vi "G2CPU Not Complex Process.vi"(10 "Backend":T1 items=["Default Backend"=0, "CPU Backend"=1, "CUDA Backend"=2, "OPENCL Backend"=4, "Intel OneAPI"=8], 11 "X size":i32=16384) -> (3 "G2CPU Time":dbl)   [LabVIEW 2020]
uses:
  <vilib>/Natan Biesmans/G2CPU GPU and CPU HPC Toolkit/ArrayFire Driver/TypeDefs/backend.ctl
  fbbaf97c-3b5e-4b4c-bc14-40c3526c788b.vi
  c2200195-6f6b-46fb-afe8-d4cd0bcb91cf.vi
  fbbaf97c-3b5e-4b4c-bc14-40c3526c788b.vi/caaf1833-0905-411b-a9ed-2cc30d41907c.vi
  <vilib>/Natan Biesmans/G2CPU GPU and CPU HPC Toolkit/G2CPU Libraries/Arrays/SubVI/Array Sizes to Dim Cluster.vi
  c2200195-6f6b-46fb-afe8-d4cd0bcb91cf.vi/caaf1833-0905-411b-a9ed-2cc30d41907c.vi
  fbbaf97c-3b5e-4b4c-bc14-40c3526c788b.vi/caaf1833-0905-411b-a9ed-2cc30d41907c.vi/1a23f98f-393f-4176-8983-7f1ab824c539.vi
  c2200195-6f6b-46fb-afe8-d4cd0bcb91cf.vi/caaf1833-0905-411b-a9ed-2cc30d41907c.vi/1a23f98f-393f-4176-8983-7f1ab824c539.vi
  <vilib>/Natan Biesmans/G2CPU GPU and CPU HPC Toolkit/G2CPU Libraries/Arrays/1DArray/f32/1D Array f32.lvclass
  C:/Program Files/National Instruments/LabVIEW 2020/vi.lib/Natan Biesmans/G2CPU GPU and CPU HPC Toolkit/G2CPU Libraries/Arrays/Array/Array Prototype.lvclass
  <vilib>/Natan Biesmans/G2CPU GPU and CPU HPC Toolkit/G2CPU Libraries/Runtime Licensing/G2CPU License Check.vi
  <vilib>/Natan Biesmans/G2CPU GPU and CPU HPC Toolkit/ArrayFire Driver/VIs/Run as Multi Device.vi
  <vilib>/Natan Biesmans/G2CPU GPU and CPU HPC Toolkit/G2CPU Libraries/Manage Environment/Find AF DLL.vi
  <vilib>/Natan Biesmans/G2CPU GPU and CPU HPC Toolkit/ArrayFire Driver/subvi/Error Converter (ErrCode or Status).vi
  <vilib>/Natan Biesmans/G2CPU GPU and CPU HPC Toolkit/G2CPU Libraries/Arrays/Array/G2CPU Set Array Pointer.vi
  <vilib>/Natan Biesmans/G2CPU GPU and CPU HPC Toolkit/G2CPU Libraries/Arrays/Array/Array Prototype.lvclass
  <vilib>/Natan Biesmans/G2CPU GPU and CPU HPC Toolkit/G2CPU Libraries/Manage Environment/G2CPU Manage Environment.lvlib
  <vilib>/Analysis/NI_AALBase.lvlib
  <vilib>/Natan Biesmans/G2CPU GPU and CPU HPC Toolkit/ArrayFire Driver/AF.lvlib
panel:
  out "imag out":dbl
  out "max value":dbl
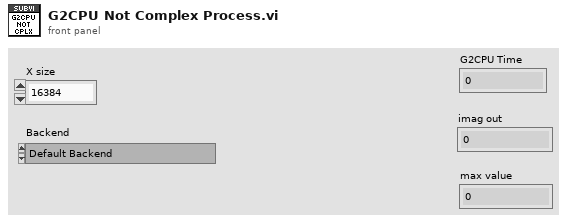
[diagram p1: front panel]
types:
  T1 = typedef "AF.lvlib/backend.ctl" = u32
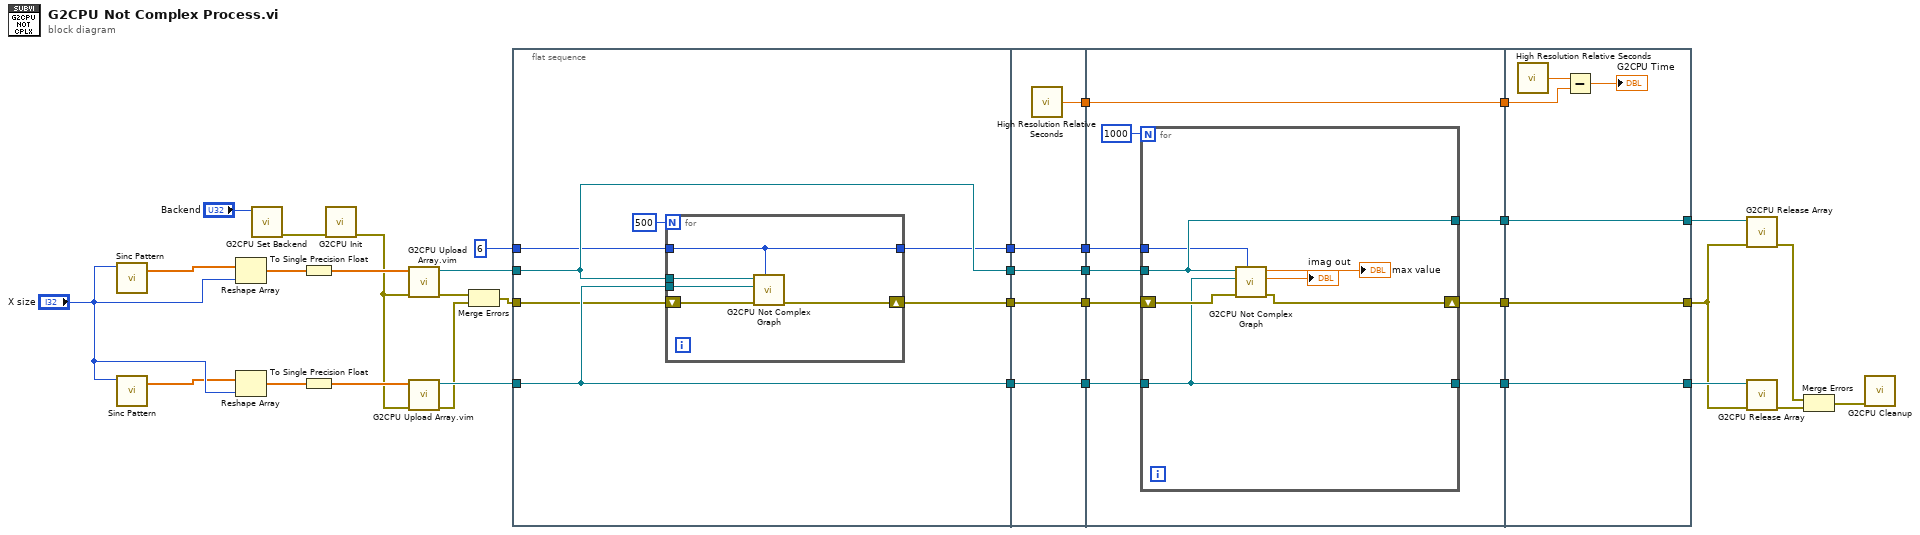
[diagram p0: block diagram]
diagram:
  n1 = call <vilib>:"Sinc Pattern.vi"("samples"="X size") -> ("Sinc Pattern"=w4:dbl[])  [unwired: 3 in, 1 out]
  n2 = call <vilib>:"Sinc Pattern.vi"("samples"="X size") -> ("Sinc Pattern"=w5:dbl[])  [unwired: 3 in, 1 out]
  n3 = Reshape Array(w4, "X size") -> (w12:dbl[])
  n4 = Reshape Array(w5, "X size") -> (w11:dbl[])
  n5 = call <vilib>:"G2CPU Set Backend.vi"("Backend"="Backend") -> ("error out"=w3:errorcluster)  [unwired: 10 in]
  n6 = To Single Precision Float(number=w12) -> (single precision float=w9:sgl[])
  n7 = To Single Precision Float(number=w11) -> (single precision float=w10:sgl[])
  n8 = call <vilib>:"G2CPU Init.vi"("error in (no error)"=w3) -> ("error out"=w1:errorcluster)  [unwired: 10 in]
  n9 = call "G2CPU Upload Array.vim"("error in (no error)"=w1, "Data"=w9) -> ("error out"=w26:errorcluster, "Array"=w30:refnum<class "1D Array f32.lvclass">)  [unwired: 8 in]
  n10 = call "G2CPU Upload Array.vim"("error in (no error)"=w1, "Data"=w10) -> ("error out"=w18:errorcluster, "Array"=w29:refnum<class "1D Array f32.lvclass">)  [unwired: 8 in]
  n11 = Merge Errors(w26, w18) -> (w19:errorcluster)
  n12 = flat-sequence {
    tunnel: w30 -> [w38]
    tunnel: [w38] -> w32
    tunnel: w29 -> [w41]
    tunnel: [w41] -> w28
    tunnel: w19 -> [w40]
    tunnel: [w42] -> w24
    tunnel: 6 ("num_loop") -> [w37]
    tunnel: [w36] -> w7
    tunnel: [w52] -> w35
    tunnel: [w51] -> w34
    tunnel: w32 -> [w51]
    tunnel: w28 -> [w50]
    tunnel: [w50] -> w27
    tunnel: [w49] -> w25
    tunnel: w24 -> [w49]
    tunnel: w7 -> [w48]
    tunnel: [w48] -> w6
    tunnel: w35 -> [w61]
    tunnel: [w61] -> w33
    tunnel: w34 -> [w60]
    tunnel: [w58] -> w31
    tunnel: w27 -> [w57]
    tunnel: w25 -> [w56]
    tunnel: [w55] -> w21
    tunnel: [w54] -> w17
    tunnel: w6 -> [w53]
    tunnel: w33 -> [w73]
    tunnel: w31 -> [w71]
    tunnel: [w71] -> w23
    tunnel: [w70] -> w22
    tunnel: w21 -> [w70]
    tunnel: [w69] -> w16
    tunnel: w17 -> [w69]
    frame #0 {
      n13 = for {
        N: 500 -> [_]
        tunnel: w38 -> [w45]
        tunnel: w41 -> [w44]
        shift-right: [w47] -> w42
        shift-left: w40 -> [w46]
        tunnel: w37 -> [w43]
        tunnel: [w43] -> w36
        n14 = call "G2CPU Not Complex Graph.vi"("num_loop"=w43, "error in (no error)"=w46, "B"=w44, "A"=w45) -> ("error out"=w47:errorcluster)  [unwired: 5 in, 2 out]
      }
    }
    frame #1 {
      n15 = call <vilib>:"High Resolution Relative Seconds.vi"() -> ("relative seconds"=w52:dbl)
    }
    frame #2 {
      n16 = for {
        N: 1000 -> [_]
        tunnel: w60 -> [w65]
        tunnel: [w65] -> w58
        tunnel: w57 -> [w64]
        tunnel: [w64] -> w55
        shift-right: [w66] -> w54
        shift-left: w56 -> [w68]
        tunnel: w53 -> [w63]
        n17 = call "G2CPU Not Complex Graph.vi"("num_loop"=w63, "error in (no error)"=w68, "B"=w64, "A"=w65) -> ("error out"=w66:errorcluster, "imag out"=→"imag out":dbl, "real out"=→"max value":dbl)  [unwired: 5 in]
      }
    }
    frame #3 {
      n18 = call <vilib>:"High Resolution Relative Seconds.vi"() -> ("relative seconds"=w74:dbl)
      n19 = Subtract(x=w74, y=w73) -> (x-y=→"G2CPU Time":dbl)
    }
  }
  n20 = call <vilib>:"G2CPU Release Array.vi"("error in (no error)"=w16, "Array in"=w23) -> ("error out"=w15:errorcluster)  [unwired: 9 in]
  n21 = call <vilib>:"G2CPU Release Array.vi"("error in (no error)"=w16, "Array in"=w22) -> ("error out"=w14:errorcluster)  [unwired: 9 in]
  n22 = Merge Errors(w15, w14) -> (w2:errorcluster)
  n23 = call <vilib>:"G2CPU Cleanup.vi"("error in (no error)"=w2) -> ()  [unwired: 10 in, 1 out]
